vi "Show.vi"(8 "error in (no error)":errorcluster, 11 "SMO.UI":refnum<class "SMO.UI.lvclass">) -> (0 "error out":errorcluster, 3 "SMO.UI out":refnum<class "SMO.UI.lvclass">)   [LabVIEW 2013, in "SMO.UI.lvclass"]
doc: "Open the front panel of the SMO.UI"
uses:
  SMO.UI.lvclass
panel:
  # "For instructions on how to use the JKI State Machine Objects, examples and video tutorials, visit:\nhttp://jki.net/state-machine-objects/\n\nJKI State Machine Objects™\nhttp://jki.net/state-machine-objects/\nCopyright (C) 2005-2015, JKI <info@jki.net>\nALL RIGHTS RESERVED"
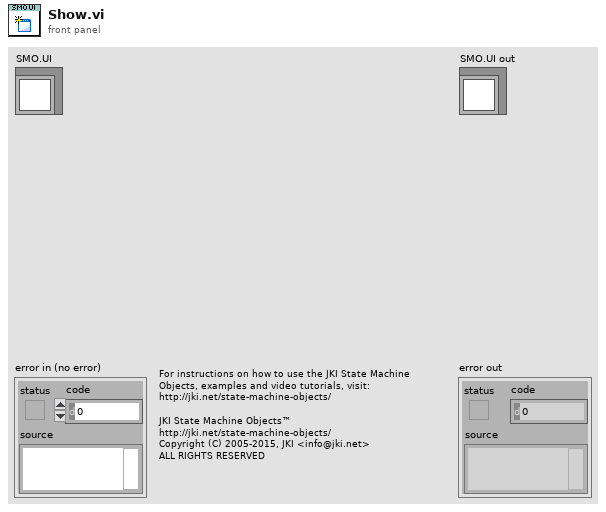
[diagram p1: front panel]
types:
  T1 = typedef "SMO.UI.lvclass/PrivateEvents--Cluster.ctl" = cluster{"Show-Hide UI":refnum<user-event>}
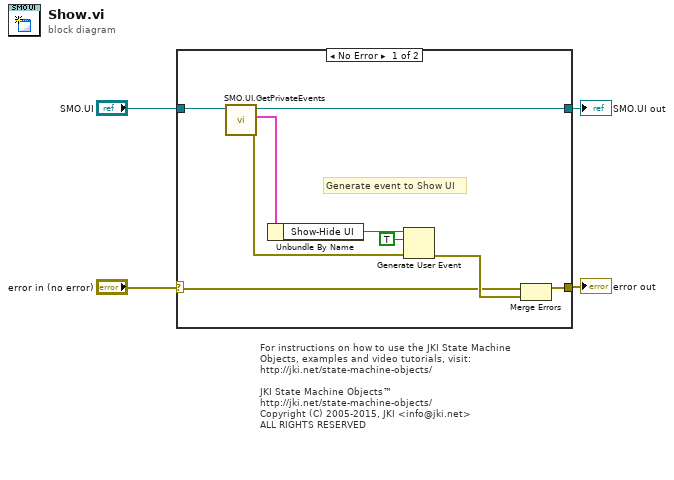
[diagram p0: block diagram]
diagram:
  # "For instructions on how to use the JKI State Machine Objects, examples and video tutorials, visit:\nhttp://jki.net/state-machine-objects/\n\nJKI State Machine Objects™\nhttp://jki.net/state-machine-objects/\nCopyright (C) 2005-2015, JKI <info@jki.net>\nALL RIGHTS RESERVED"
  n1 = case shown="No Error" "error in (no error)" {
    selector: "error in (no error)" -> [w5 w15]
    tunnel: "SMO.UI" -> [w6 w14]
    tunnel: [w13 w15] -> w3
    tunnel: [w11 w14] -> w2
    frame No Error {
      # "Generate event to Show UI"
      n2 = call "SMO.UI.GetPrivateEvents.vi"("SMO.UI"=w6) -> ("error out"=w10:errorcluster, "SMO.UI Private Events"=w8:T1, "SMO.UI out"=w11:refnum<class "SMO.UI.lvclass">)  [unwired: 8 in]
      n3 = Unbundle By Name(w8) -> ("Show-Hide UI"=w9:refnum<user-event>)
      n4 = Generate User Event(user event=w9, event data cluster=TRUE ("event data"), error in=w10) -> (error out=w12:errorcluster)  [unwired: 1 in, 1 out]
      n5 = Merge Errors(w5, w12) -> (w13:errorcluster)
    }
    frame Error {
    }
  }
  "error out" <- w3
  "SMO.UI out" <- w2
